vi "initi_config.vi"(8 "error in (no error)":errorcluster, 11 "config_file_name":string="reg_service_config.ini") -> (0 "error out":errorcluster, 3 "Cfg Data":T1)   [LabVIEW 2015]
uses:
  typedef/init_config_data.ctl
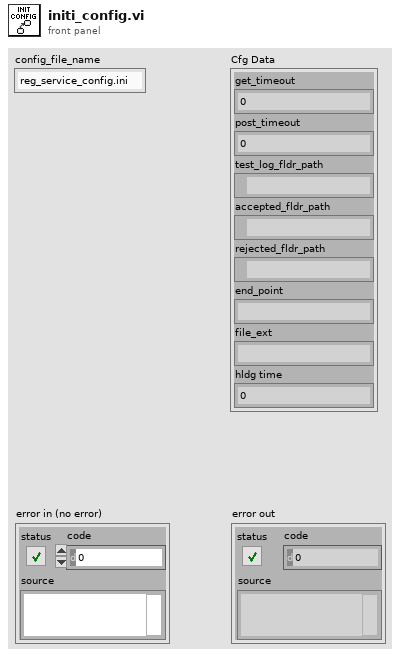
[diagram p1: front panel]
types:
  T1 = typedef "init_config_data.ctl" = cluster{"end_point":string, "file_ext":string, "hldg time":dbl, "test_log_fldr_path":path, "accepted_fldr_path":path, "rejected_fldr_path":path, "post_timeout":i32, "get_timeout":i32}
  T2 = cluster{"test_log_base_path":string, "accepted_folder_name":string, "rejected_folder_name":string}
  T3 = typedef "created_folders_path.ctl" = cluster{"test_log_fldr_path":path, "accepted_fldr_path":path, "rejected_fldr_path":path}
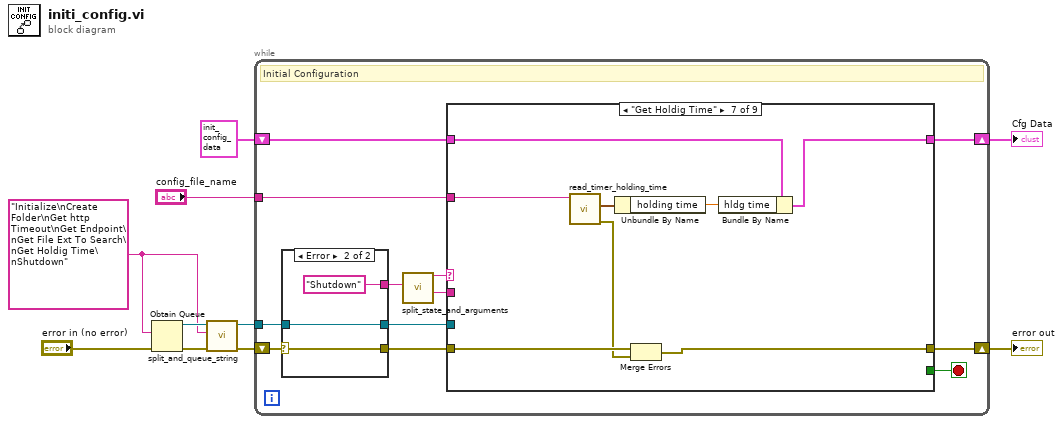
[diagram p0: block diagram]
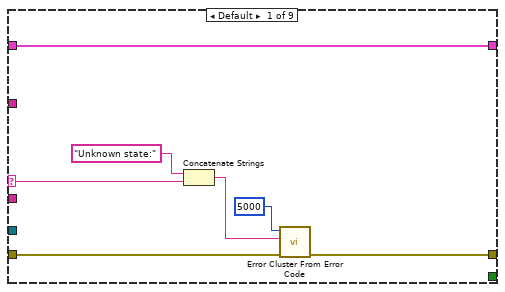
[diagram p2: hidden frame]
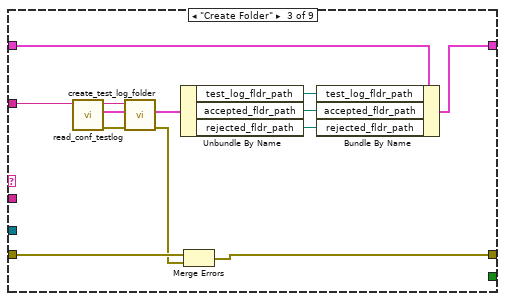
[diagram p4: hidden frame]
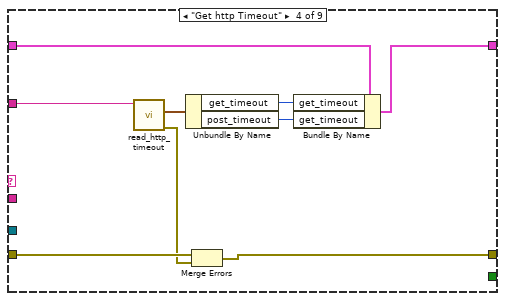
[diagram p5: hidden frame]
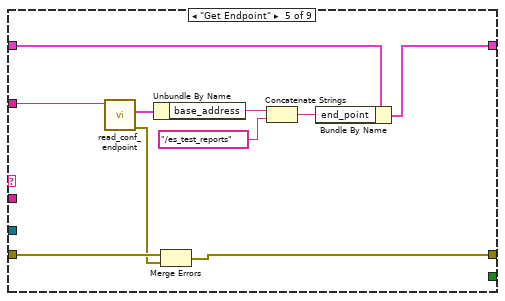
[diagram p6: hidden frame]
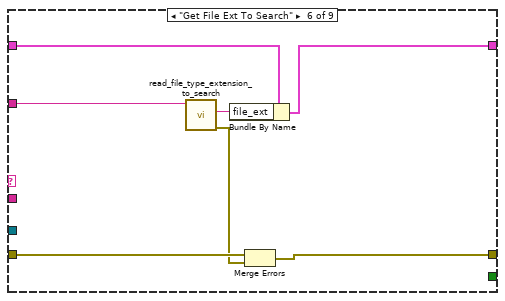
[diagram p7: hidden frame]
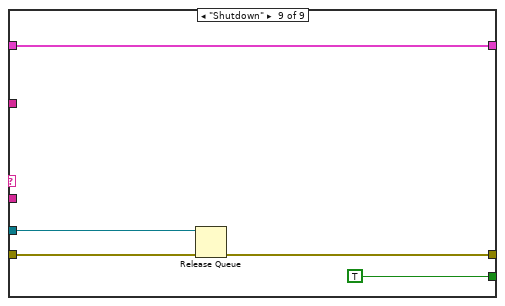
[diagram p9: hidden frame]
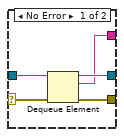
[diagram p10: hidden frame]
diagram:
  w6 = "Initialize\nCreate Folder\nGet http Timeout\nGet Endpoint\nGet File Ext To Search\nGet Holdig Time\nShutdown"
  n1 = Obtain Queue(element data type=w6, error in (no error)="error in (no error)") -> (queue out=w10:refnum<queue>, error out=w9:errorcluster)  [unwired: 3 in, 1 out]
  n2 = call "split_and_queue_string.vi"("error in (no error)"=w9, "program string"=w6, "queue in"=w10) -> ("error out"=w8:errorcluster, "queue out"=w7:refnum<queue>)  [unwired: 7 in]
  n3 = while {
    shift-right: [w20] -> w4
    shift-left: w8 -> [w22]
    tunnel: w7 -> [w18]
    shift-right: [w12] -> w2
    shift-left: T1 {"end_point"="", "file_ext"="", "hldg time"=0.0, "test_log_fldr_path"=path "", "accepted_fldr_path"=path "", "rejected_fldr_path"=path "", "post_timeout"=0, "get_timeout"=0} ("Data") -> [w13]
    tunnel: "config_file_name" -> [w11]
    stop <- w19 stop-if-true
    # "Initial Configuration"
    n4 = case shown="Error" w22 {
      selector: w22 -> [w90 w93]
      tunnel: [w89 w93] -> w21
      tunnel: w18 -> [w88 w92]
      tunnel: [w87 w92] -> w17
      tunnel: [w86 "Shutdown"] -> w14
      frame No Error {
        n5 = Dequeue Element(queue=w88, error in (no error)=w90) -> (queue out=w87:refnum<queue>, element=w86:string, error out=w89:errorcluster)  [unwired: 1 in, 1 out]
      }
      frame Error {
      }
    }
    n6 = call "split_state_and_arguments.vi"("String"=w14) -> ("Arguments"=w15:string, "State"=w16:string)  [unwired: 9 in]
    n7 = case shown="\"Get Holdig Time\"" w16 {
      selector: w16 -> [w28 _ _ _ _ _ _ _ _]
      tunnel: w21 -> [w27 w31 w44 w53 w63 w70 w78 w80 w84]
      tunnel: [w26 w31 w37 w49 w55 w67 w73 w80 w82] -> w20
      tunnel: [_ _ _ _ _ _ _ _ TRUE] -> w19
      tunnel: w17 -> [_ _ _ _ _ _ _ _ w83]
      tunnel: w15 -> [_ _ _ _ _ _ _ _ _]
      tunnel: w11 -> [_ _ w40 w52 w58 w68 w75 _ _]
      tunnel: w13 -> [w23 w30 w39 w51 w57 w65 w74 w79 w81]
      tunnel: [w23 w30 w38 w50 w56 w64 w71 w79 w81] -> w12
      frame Default {
        n8 = Concatenate Strings("Unknown state:", w28) -> (w25:string)
        n9 = call <vilib>:"Error Cluster From Error Code.vi"("error in (no error)"=w27, "error message (\"\")"=w25, "error code (0)"=5000) -> ("error out"=w26:errorcluster)  [unwired: 6 in]
      }
      frame "Initialize" {
      }
      frame "Create Folder" {
        n10 = call "read_conf_testlog.vi"("config_file_name"=w40) -> ("error out"=w43:errorcluster, "values"=w42:T2, "config_file_name_out"=w41:string)  [unwired: 8 in]
        n11 = call "create_test_log_folder.vi"("error in (no error)"=w43, "names in"=w42, "config_file_name"=w41) -> ("error out"=w36:errorcluster, "foldr paths"=w35:T3)  [unwired: 6 in, 1 out]
        n12 = Unbundle By Name(w35) -> ("test_log_fldr_path"=w34:path, "accepted_fldr_path"=w33:path, "rejected_fldr_path"=w32:path)
        n13 = Merge Errors(w44, w36) -> (w37:errorcluster)
        n14 = Bundle By Name(cluster=w39, "test_log_fldr_path"=w34, "accepted_fldr_path"=w33, "rejected_fldr_path"=w32) -> (w38:T1)
      }
      frame "Get http Timeout" {
        n15 = call "read_http_timeout.vi"("config_file_name"=w52) -> ("error out"=w48:errorcluster, "values"=w47:cluster{"get_timeout":i32, "post_timeout":i32})  [unwired: 8 in, 1 out]
        n16 = Unbundle By Name(w47) -> ("get_timeout"=w46:i32, "post_timeout"=w45:i32)
        n17 = Merge Errors(w53, w48) -> (w49:errorcluster)
        n18 = Bundle By Name(cluster=w51, "get_timeout"=w46, "get_timeout"=w45) -> (w50:T1)
      }
      frame "Get Endpoint" {
        n19 = call "read_conf_endpoint.vi"("config_file_name"=w58) -> ("error out"=w54:errorcluster, "values"=w59:cluster{"base_address":string})  [unwired: 8 in, 1 out]
        n20 = Unbundle By Name(w59) -> ("base_address"=w60:string)
        n21 = Merge Errors(w63, w54) -> (w55:errorcluster)
        n22 = Concatenate Strings(w60, "/es_test_reports" ("string")) -> (w62:string)
        n23 = Bundle By Name(cluster=w57, "end_point"=w62) -> (w56:T1)
      }
      frame "Get File Ext To Search" {
        n24 = call "read_file_type_extension_to_search.vi"("config_file_name"=w68) -> ("error out"=w66:errorcluster, "extension_to_search"=w69:string)  [unwired: 8 in, 1 out]
        n25 = Bundle By Name(cluster=w65, "file_ext"=w69) -> (w64:T1)
        n26 = Merge Errors(w70, w66) -> (w67:errorcluster)
      }
      frame "Get Holdig Time" {
        n27 = call "read_timer_holding_time.vi"("config_file_name"=w75) -> ("error out"=w72:errorcluster, "values"=w76:cluster{"holding time":dbl})  [unwired: 8 in, 1 out]
        n28 = Unbundle By Name(w76) -> ("holding time"=w77:dbl)
        n29 = Merge Errors(w78, w72) -> (w73:errorcluster)
        n30 = Bundle By Name(cluster=w74, "hldg time"=w77) -> (w71:T1)
      }
      frame "Idle" {
      }
      frame "Shutdown" {
        n31 = Release Queue(queue=w83, error in (no error)=w84) -> (error out=w82:errorcluster)  [unwired: 1 in, 2 out]
      }
    }
  }
  "error out" <- w4
  "Cfg Data" <- w2
